vi "Parse Empty Tag.vi"(8 "Error In":errorcluster) -> (0 "Error Out":errorcluster)   [LabVIEW 2017, in "Tests.lvlib" / "Parser.lvlib"]
uses:
  Parser.lvlib
  src/Mustache/Public/Tokens/Public/EscapedVariable/EscapedVariable.lvclass
  src/Mustache/Public/Tokens/Public/EscapedVariable/EscapedVariable.lvclass/EscapedVariable.ctl
  src/Mustache/Public/Readers/Public/String/String.lvclass
  D:/Users/cfield/Code/Field R&D Services/Mustache/feature-lv-original-parser/src/Mustache/Public/Readers/Public/Abstract/Abstract.lvclass
  <vilib>/addons/_JKI Toolkits/Caraya/classes/Test/Test.lvclass
  src/Mustache/Public/Parser/Parser.lvclass
  <vilib>/addons/_JKI Toolkits/Caraya/classes/Assert/Assert.lvclass
  src/Mustache/Public/Tokens/Public/Abstract/Abstract.lvclass
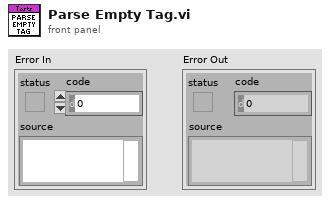
[diagram p1: front panel]
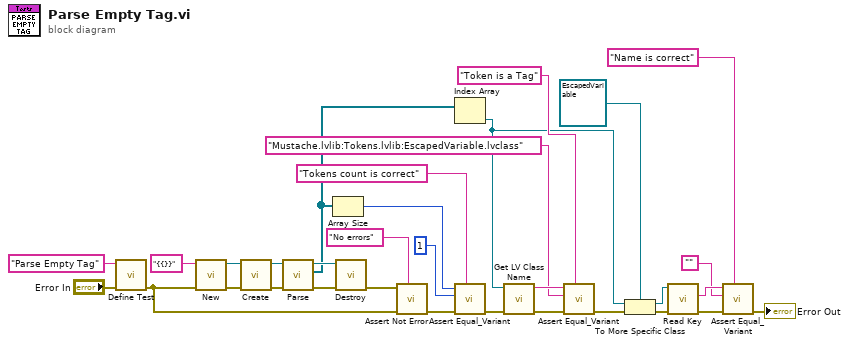
[diagram p0: block diagram]
diagram:
  n1 = call <vilib>:"Define Test.vi"("error in (no error)"="Error In", "Label (VI Title)"="Parse Empty Tag") -> ("error out"=w23:errorcluster)  [unwired: 9 in]
  n2 = call "New.vi"("Error In"=w23, "String"="{{}}") -> ("Error Out"=w29:errorcluster, "String"=w30:refnum<class "String.lvclass">)  [unwired: 8 in]
  n3 = call "Create.vi"("Error In"=w29, "Reader"=w30) -> ("Error Out"=w28:errorcluster, "Parser"=w27:refnum<class "Parser.lvclass">)  [unwired: 8 in]
  n4 = call "Parse.vi"("Error In"=w28, "Parser In"=w27) -> ("Error Out"=w25:errorcluster, "Tokens"=w17:refnum<class "Abstract.lvclass">[], "Parser Out"=w26:refnum<class "Parser.lvclass">)  [unwired: 7 in]
  n5 = Array Size(array=w17) -> (size(s)=w19:i32)
  n6 = call "Destroy.vi"("Error In"=w25, "Parser"=w26) -> ("Error Out"=w24:errorcluster)  [unwired: 9 in]
  n7 = call <vilib>:"Assert Not Error.vi"("Label"="No errors", "error in (no error)"=w23, "Not Error?"=w24) -> ("error out"=w21:errorcluster)  [unwired: 8 in]
  n8 = Index Array(array=w17) -> (element=w10:refnum<class "Abstract.lvclass">)  [unwired: 1 in]
  n9 = call <vilib>:"Assert Equal_Variant.vi"("Label"="Tokens count is correct", "error in (no error)"=w21, "Y"=1 ("size(s)"), "X"=w19) -> ("error out"=w15:errorcluster)  [unwired: 7 in]
  n10 = call <vilib>:"Get LV Class Name.vi"("error in (no error)"=w15, "object"=w10) -> ("error out"=w14:errorcluster, "class name"=w13:string)  [unwired: 8 in]
  n11 = call <vilib>:"Assert Equal_Variant.vi"("Label"="Token is a Tag", "error in (no error)"=w14, "Y"="Mustache.lvlib:Tokens.lvlib:EscapedVariable.lvclass", "X"=w13) -> ("error out"=w11:errorcluster)  [unwired: 7 in]
  n12 = To More Specific Class(target class=refnum<class "EscapedVariable.lvclass"> refnum ("Mustache.lvlib:Tokens.lvlib:Tag.lvclass"), reference=w10, error in=w11) -> (specific class reference=w7:refnum<class "EscapedVariable.lvclass">, error out=w8:errorcluster)
  n13 = call "Read Key.vi"("Error In"=w8, "Tag In"=w7) -> ("Error Out"=w4:errorcluster, "Key"=w5:string)  [unwired: 7 in, 1 out]
  n14 = call <vilib>:"Assert Equal_Variant.vi"("Label"="Name is correct", "error in (no error)"=w4, "Y"="", "X"=w5) -> ("error out"=→"Error Out":errorcluster)  [unwired: 7 in]
